vi "Initialize Page Number.vi"(8 "error in (no error)":errorcluster, 11 "Project Model in":refnum<class "Project Model.lvclass">) -> (0 "error out":errorcluster, 3 "Project Model out":refnum<class "Project Model.lvclass">)   [LabVIEW 2013, in "Project Model.lvlib" / "Project Model.lvclass"]
uses:
  Project Model.lvclass
  Project Model.lvclass/Project Model.ctl
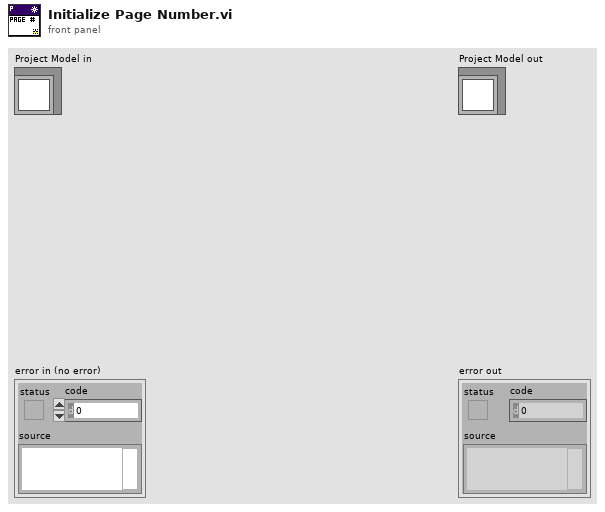
[diagram p1: front panel]
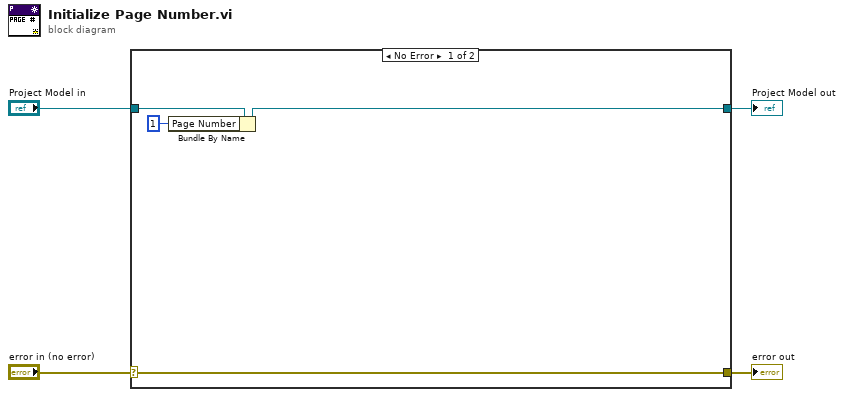
[diagram p0: block diagram]
diagram:
  n1 = case shown="No Error" "error in (no error)" {
    selector: "error in (no error)" -> [w7 w10]
    tunnel: [w7 w10] -> w3
    tunnel: [w6 w9] -> w1
    tunnel: "Project Model in" -> [w8 w9]
    frame No Error {
      n2 = Bundle By Name(cluster=w8, "Page Number"=1) -> (w6:refnum<class "Project Model.lvclass">)
    }
    frame Error {
    }
  }
  "error out" <- w3
  "Project Model out" <- w1
